vi "lv_list.vi"   [LabVIEW 2020]
doc: "G-CLI tool to list installed LabView development versions.s"
uses:
  <vilib>/Wiresmith Technology/G CLI/Argument Parser/Option Class/Option Configuration.ctl
  <vilib>/Wiresmith Technology/G CLI/Argument Parser/Option Class/Argument Type.ctl
  <vilib>/Utility/error.llb/DialogType.ctl
  094f6021-4ef8-4573-82ce-a7b4949f6c5c.vi
  67a138f0-9744-4b2d-9c21-223ad79f4533.vi
  6795289f-0a04-455c-a499-a5e59a361415.vi
  <vilib>/JDP Science/JSONtext/Variant to JSON Text.vi
  <vilib>/JDP Science/JSONtext/LVClass Serializer/JSONtext LVClass Serializer.lvclass
  <vilib>/regexp/Match Regular Expression.xnode
  <vilib>/Wiresmith Technology/G CLI/CLI Class/CLI.lvclass
  <vilib>/Wiresmith Technology/G CLI/Argument Parser/Option Set Class/Option Set.lvclass
  <vilib>/Wiresmith Technology/G CLI/Argument Parser/Option Class/Option.lvclass
  <vilib>/JDP Science/JSONtext/JSONtext.lvlib
types:
  T1 = cluster{"VerboseMode":bool, "JsonOutput":bool, "ShortOutput":bool}
  T2 = enum32{"Invalid", "Standard", "Closed", "Hidden", "Minimized", "Maximized"}
  T3 = typedef "Option Parser.lvlib/Option.lvclass/Option Configuration.ctl" = cluster{"Option Type":T4, "Option Labels":string[], "Key":string, "Description":string, "Required":bool, "Default Value":string}
  T4 = typedef "Option Parser.lvlib/Option.lvclass/Argument Type.ctl" = enum16{"flag", "value"}
  T5 = typedef "LabViewApplication--cluster.ctl" = cluster{"Bitness":enum8{"Unknown", "x86", "x64"}, "Version":string, "LabVIEW.exe":path, "VersionString":string}
  T6 = typedef "DialogType.ctl" = u16
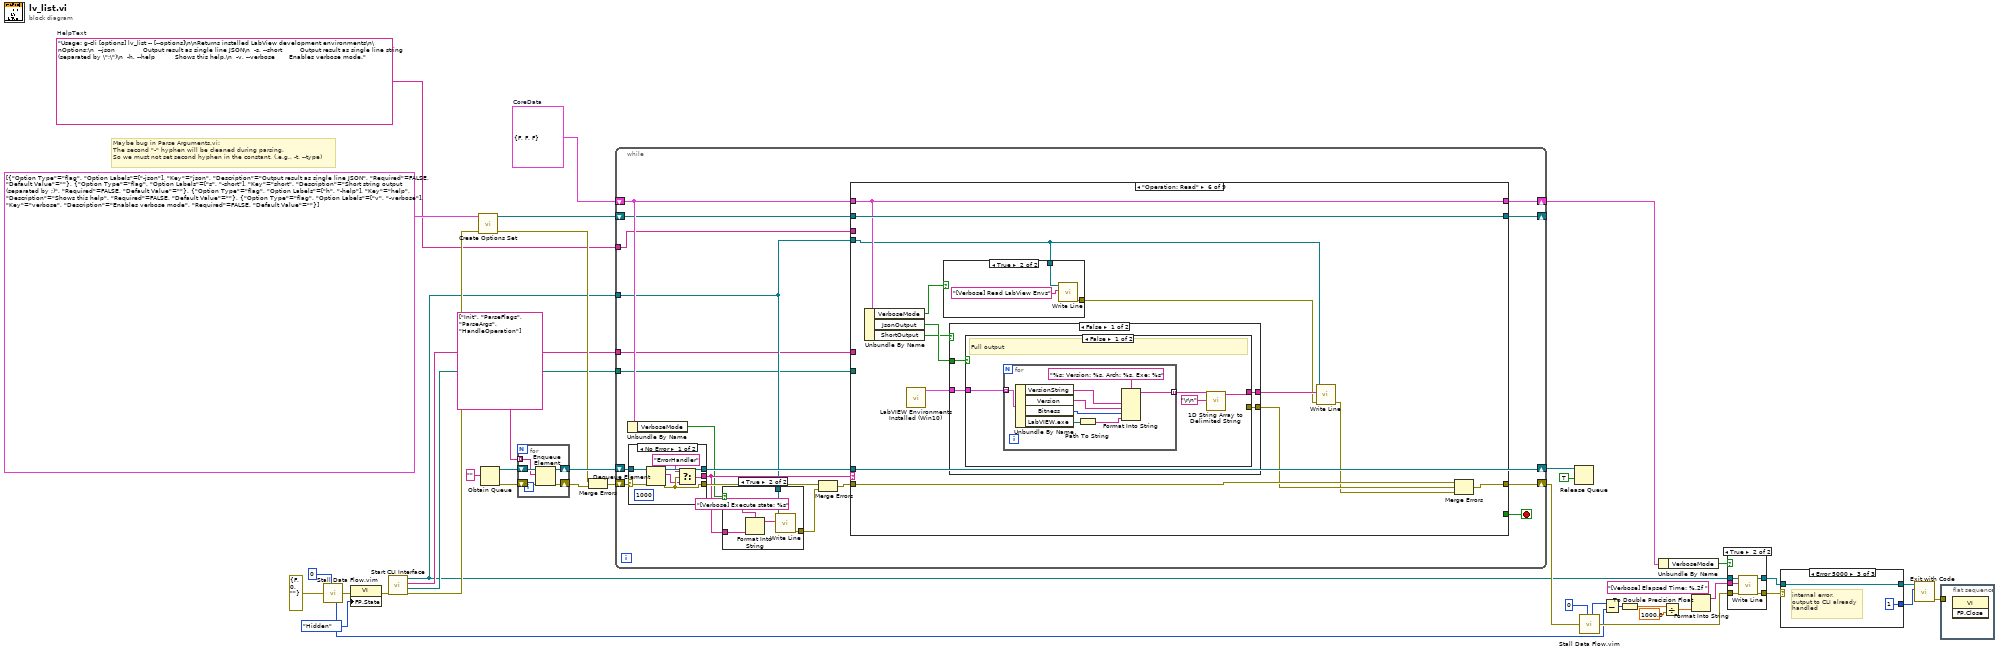
[diagram p0: block diagram]
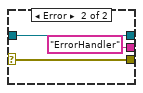
[diagram p4: hidden frame]
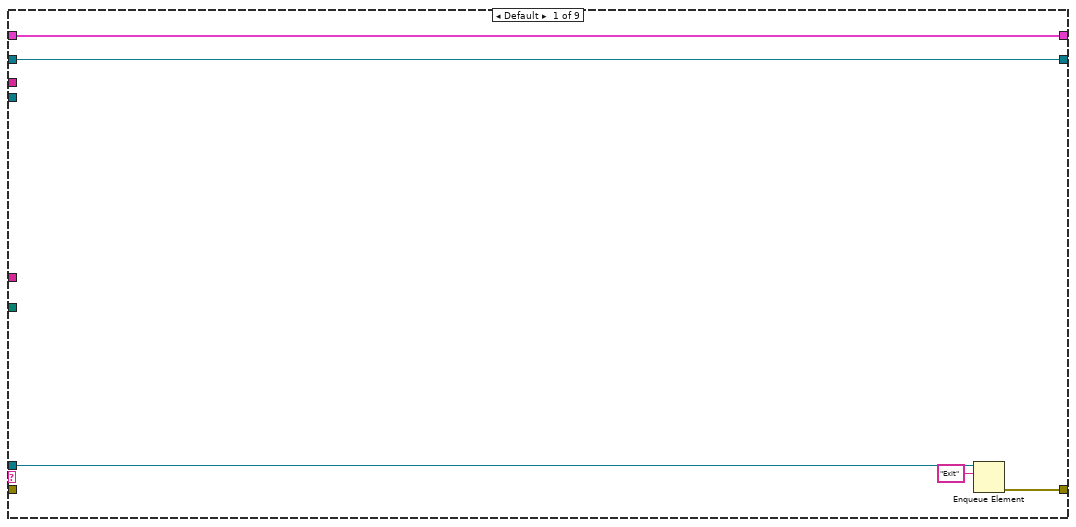
[diagram p5: hidden frame]
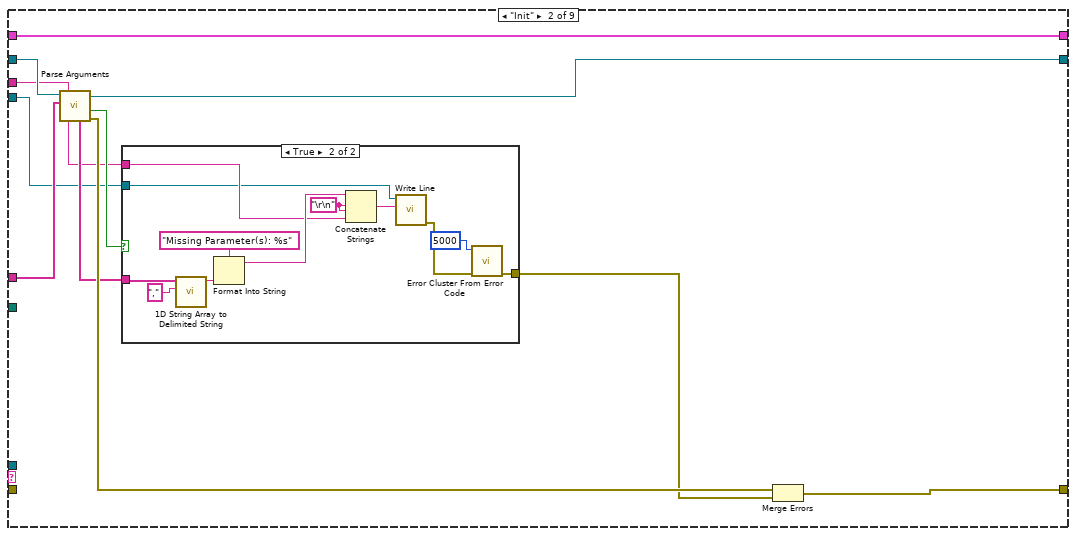
[diagram p6: hidden frame]
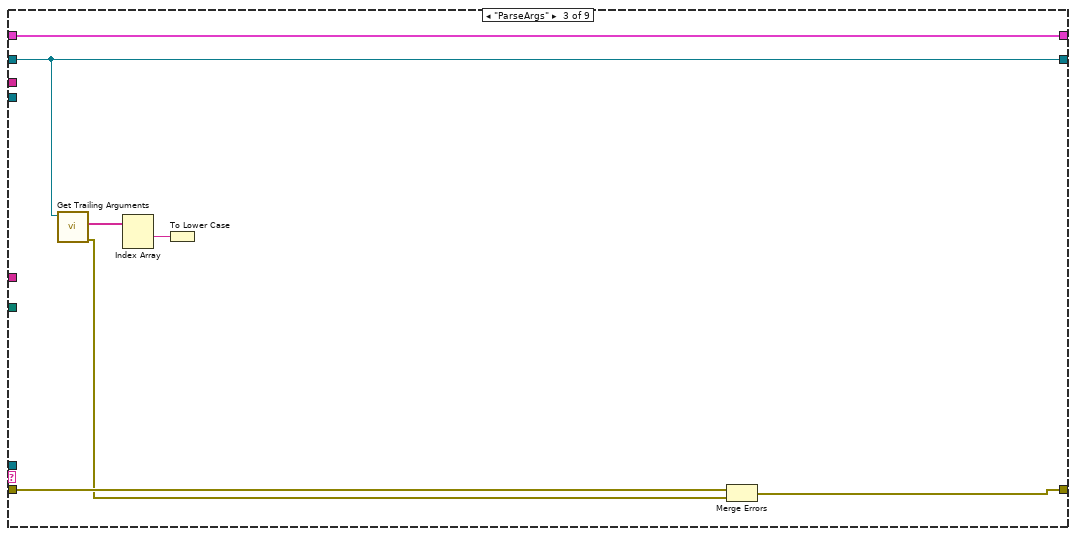
[diagram p8: hidden frame]
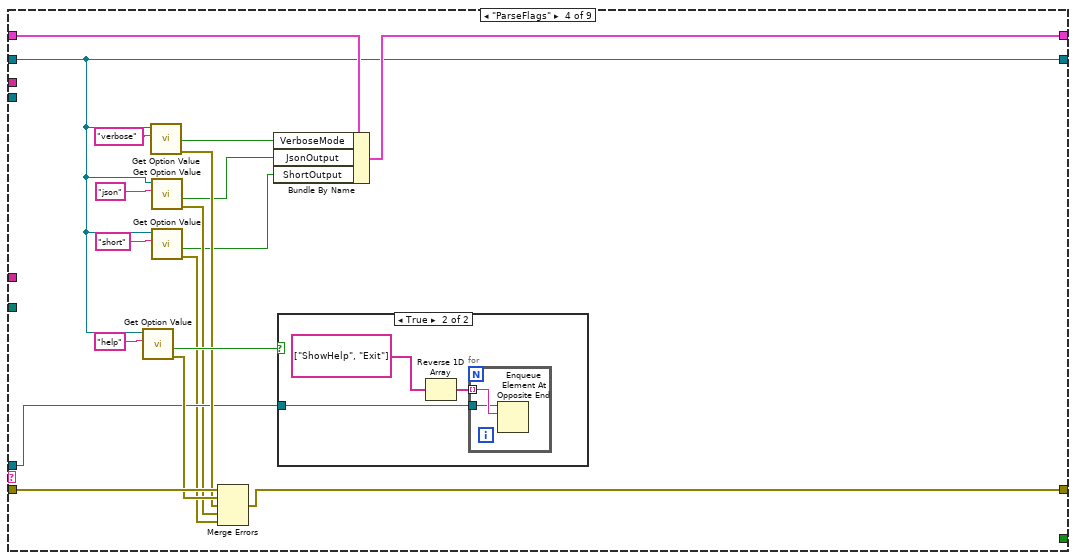
[diagram p9: hidden frame]
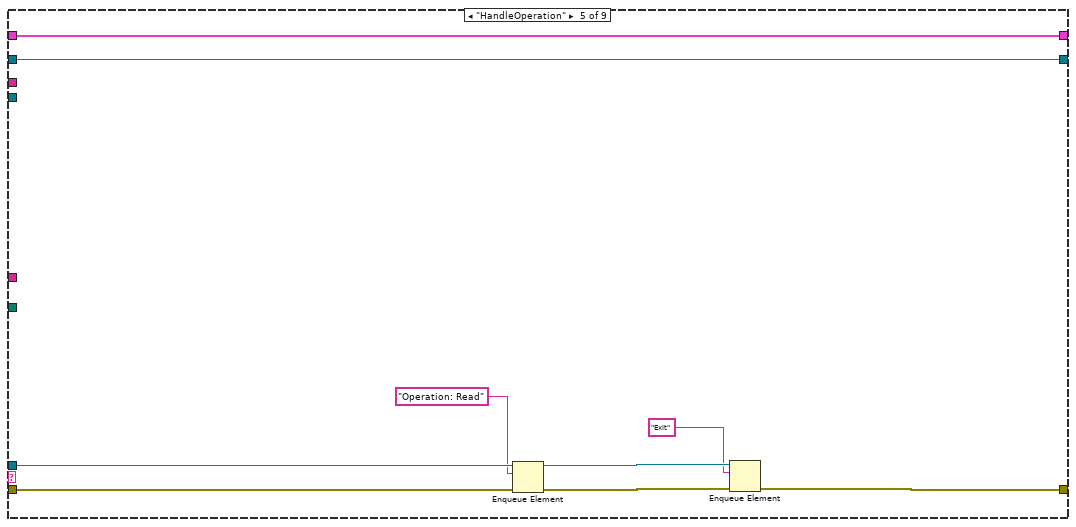
[diagram p11: hidden frame]
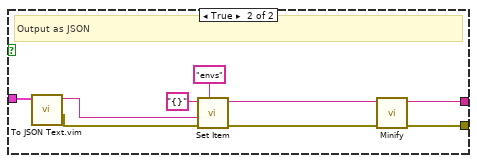
[diagram p12: hidden frame]
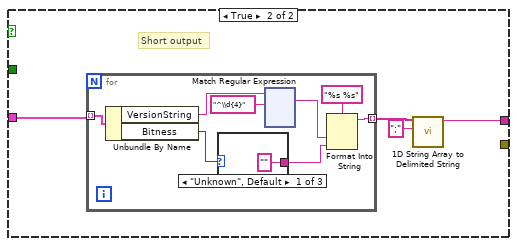
[diagram p13: hidden frame]
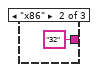
[diagram p14: hidden frame]
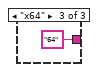
[diagram p15: hidden frame]
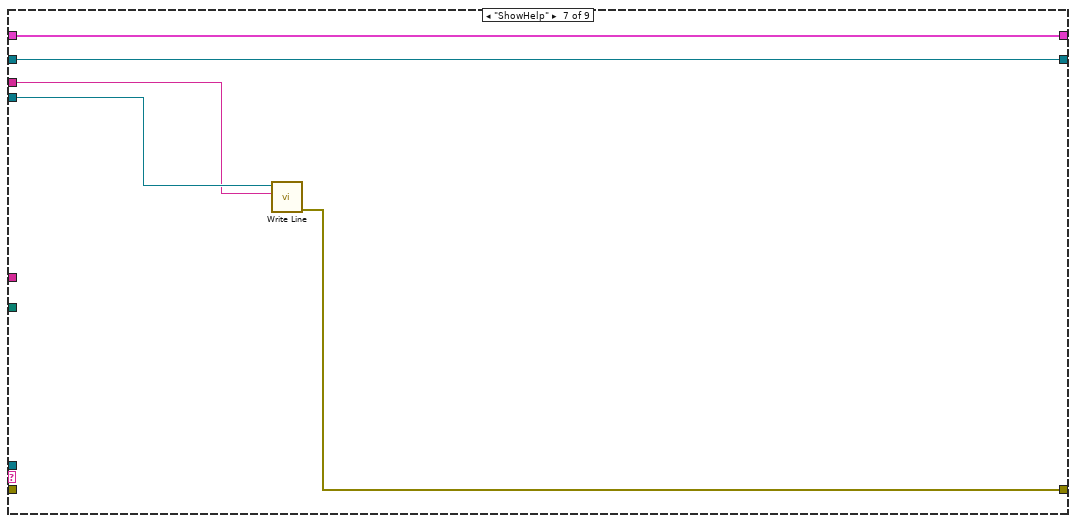
[diagram p17: hidden frame]
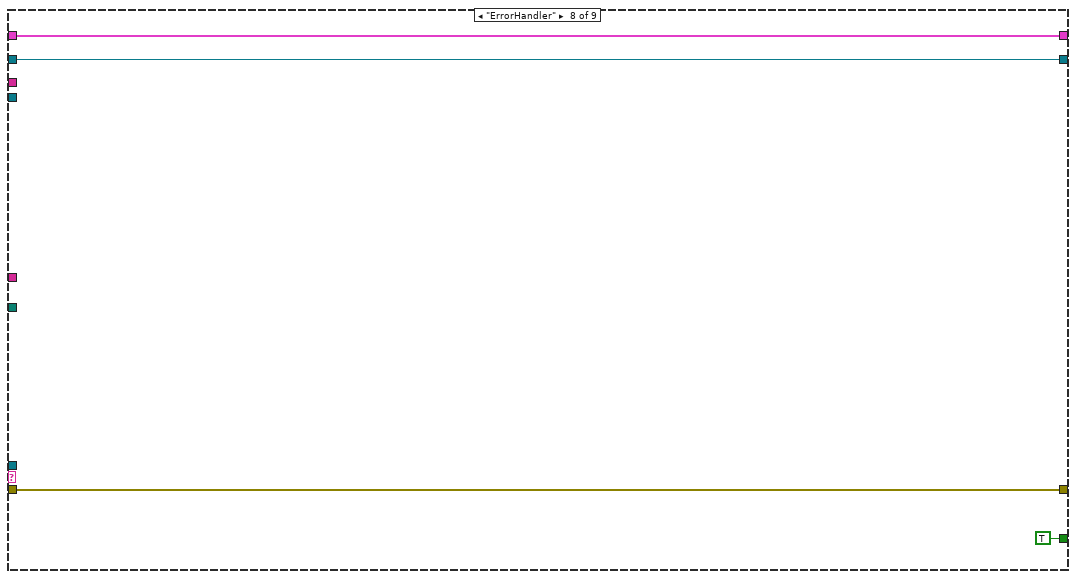
[diagram p18: hidden frame]
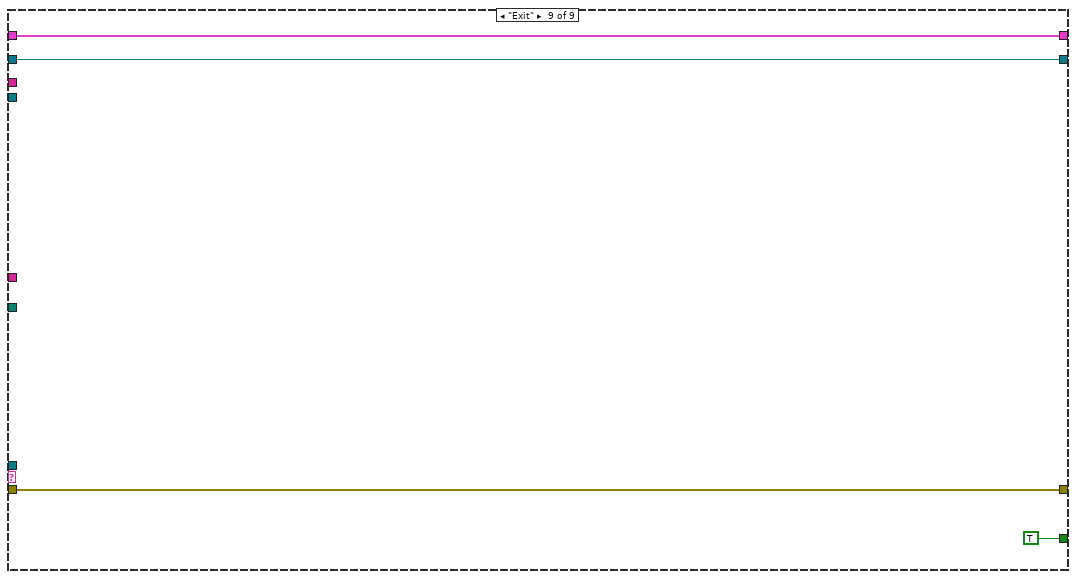
[diagram p19: hidden frame]
diagram:
  w1 = "Usage: g-cli [options] lv_list -- [--options]\n\nReturns installed LabView development environments\n\nOptions:\n  --json              Output result as single line JSON\n  -s, --short         Output result as single line string (separated by \";\")\n  -h, --help          Shows this help.\n  -v, --verbose       Enables verbose mode."  # HelpText
  w14 = T1 {"VerboseMode"=FALSE, "JsonOutput"=FALSE, "ShortOutput"=FALSE}  # CoreData
  # "Maybe bug in Parse Arguments.vi: \nThe second \"-\" hyphen will be cleaned during parsing.\nSo we must not set second hyphen in the constant. (.e.g., -t, --type)"
  n1 = call "Stall Data Flow.vim"("value in"=errorcluster {"status"=FALSE, "code"=0, "source"=""} ("error in (no error)"), "milliseconds to wait"=u32 0) -> ("millisecond timer value"=w30:u32, "value out"=w37:errorcluster)
  n2 = property class="VI"(error in=w37, "FP.State"=T2."Hidden" ("Front Panel Window:State")) -> (error out=w36:errorcluster)  [unwired: 1 in, 1 out]
  n3 = call <vilib>:"Start CLI Interface.vi"("error in (no error)"=w36) -> ("error out"=w41:errorcluster, "Working Directory"=w7:path, "Custom Parameters"=w8:string[], "CLI out"=w5:refnum<class "CLI.lvclass">)  [unwired: 7 in]
  n4 = call <vilib>:"Create Options Set.vi"("error in (no error)"=w41, "Options"=T3[] [{"Option Type"=enum."flag", "Option Labels"=["-json"], "Key"="json", "Description"="Output result as single line JSON", "Required"=FALSE, "Default Value"=""}, {"Option Type"=enum."flag", "Option Labels"=["s", "-short"], "Key"="short", "Description"="Short string output (separated by ;)", "Required"=FALSE, "Default Value"=""}, {"Option Type"=enum."flag", "Option Labels"=["h", "-help"], "Key"="help", "Description"="Shows this help", "Required"=FALSE, "Default Value"=""}, {"Option Type"=enum."flag", "Option Labels"=["v", "-verbose"], "Key"="verbose", "Description"="Enables verbose mode", "Required"=FALSE, "Default Value"=""}]) -> ("error out"=w10:errorcluster, "Option Set out"=w12:refnum<class "Option Set.lvclass">)  [unwired: 8 in]
  n5 = Obtain Queue(element data type="") -> (queue out=w19:refnum<queue>, error out=w16:errorcluster)  [unwired: 4 in, 1 out]
  n6 = for {
    shift-right: [w45] -> w17
    shift-left: w19 -> [w46]
    shift-right: [w43] -> w11
    shift-left: w16 -> [w44]
    tunnel: string[] ["Init", "ParseFlags", "ParseArgs", "HandleOperation"] -> [w42] mode=indexing
    n7 = Enqueue Element(queue=w46, element=w42, error in (no error)=w44) -> (queue out=w45:refnum<queue>, error out=w43:errorcluster)  [unwired: 1 in, 1 out]
  }
  n8 = Merge Errors(w10, w11) -> (w9:errorcluster)
  n9 = while {
    shift-right: [w61] -> w4
    shift-left: w14 -> [w56]
    shift-right: [w59] -> w6
    shift-left: w9 -> [w63]
    shift-right: [w58] -> w15
    shift-left: w17 -> [w64]
    tunnel: w5 -> [w54]
    tunnel: w8 -> [w49]
    tunnel: w7 -> [w50]
    tunnel: w1 -> [w48]
    shift-right: [w47] -> _
    shift-left: w12 -> [w53]
    stop <- w60 stop-if-true
    n10 = Unbundle By Name(w56) -> ("VerboseMode"=w55:bool)
    n11 = case shown="No Error" w63 {
      selector: w63 -> [w75 w79]
      tunnel: w64 -> [w76 w78]
      tunnel: [w71 "ErrorHandler"] -> w57
      tunnel: [w73 w79] -> w62
      tunnel: [w74 w78] -> w58
      frame No Error {
        (unwired) 1000 ("timeout in ms (-1)")
        n12 = Dequeue Element(queue=w76, error in (no error)=w75) -> (queue out=w74:refnum<queue>, element=w72:string, error out=w73:errorcluster)  [unwired: 1 in, 1 out]
        n13 = Select(t="ErrorHandler", s=w73, f=w72) -> (s? t:f=w71:string)
      }
      frame Error {
      }
    }
    n14 = case shown="True" w55 {
      tunnel: w57 -> [_ w69]
      tunnel: w54 -> [_ w66]
      tunnel: [_ w65] -> w51
      frame False {
      }
      frame True {
        n15 = Format Into String(format string="[Verbose] Execute state: %s", w69) -> (resulting string=w67:string)  [unwired: 2 in, 1 out]
        n16 = call <vilib>:"Write Line.vi"("Text to Write"=w67, "CLI in"=w66) -> ("error out"=w65:errorcluster)  [unwired: 8 in, 1 out]
      }
    }
    n17 = Merge Errors(w62, w51) -> (w52:errorcluster)
    n18 = case shown="\"Operation: Read\"" w57 {
      tunnel: w52 -> [_ _ w113 w129 w144 w157 _ w324 w327]
      tunnel: [w84 w95 w114 w122 w145 w158 w321 w325 w329] -> w61
      tunnel: w56 -> [w84 w95 w114 w132 w145 w158 w321 w325 w329]
      tunnel: [_ _ _ _ _ _ _ TRUE TRUE] -> w60
      tunnel: [w82 w87 w109 w127 w139 w156 w317 w324 w327] -> w59
      tunnel: w58 -> [w83 _ _ w123 w143 _ _ _ _]
      tunnel: w54 -> [_ w88 _ _ _ w154 w319 _ _]
      tunnel: w53 -> [w80 w94 w112 w117 w146 w159 w320 w322 w326]
      tunnel: w50 -> [_ _ _ _ _ _ _ _ _]
      tunnel: w49 -> [_ w93 _ _ _ _ _ _ _]
      tunnel: w48 -> [_ w89 _ _ _ _ w318 _ _]
      tunnel: [w80 w85 w112 w117 w146 w159 w320 w322 w326] -> w47
      frame Default {
        n19 = Enqueue Element(queue=w83, element="Exit") -> (error out=w82:errorcluster)  [unwired: 2 in, 2 out]
      }
      frame "Init" {
        n20 = call <vilib>:"Parse Arguments.vi"("Arguments"=w93, "Option Set in"=w94) -> ("error out"=w92:errorcluster, "Missing Options"=w91:bool, "Option Set out"=w85:refnum<class "Option Set.lvclass">, "Missing Option Keys"=w90:string[])  [unwired: 6 in]
        n21 = case shown="True" w91 {
          tunnel: w90 -> [_ w106]
          tunnel: w89 -> [_ w101]
          tunnel: w88 -> [_ w99]
          tunnel: [_ w96] -> w86
          frame False {
          }
          frame True {
            w103 = "\r\n"
            n22 = call <vilib>:"1D String Array to Delimited String.vi"("delimiter"=",", "string array"=w106) -> ("delimited string"=w104:string)  [unwired: 9 in]
            n23 = Format Into String(format string="Missing Parameter(s): %s", w104) -> (resulting string=w102:string)  [unwired: 2 in, 1 out]
            n24 = Concatenate Strings(w102, w103, w103, w101) -> (w100:string)
            n25 = call <vilib>:"Write Line.vi"("Text to Write"=w100, "CLI in"=w99) -> ("error out"=w97:errorcluster)  [unwired: 8 in, 1 out]
            n26 = call <vilib>:"Error Cluster From Error Code.vi"("error in (no error)"=w97, "error code (0)"=5000) -> ("error out"=w96:errorcluster)  [unwired: 7 in]
          }
        }
        n27 = Merge Errors(w92, w86) -> (w87:errorcluster)
      }
      frame "ParseArgs" {
        n28 = call <vilib>:"Get Trailing Arguments.vi"("Option Set in"=w112) -> ("error out"=w108:errorcluster, "Arguments"=w111:string[])  [unwired: 8 in, 1 out]
        n29 = Index Array(array=w111) -> (element #1=w110:string)  [unwired: 2 in, 1 out]
        n30 = To Lower Case(string=w110) -> ()  [unwired: 1 out]
        n31 = Merge Errors(w113, w108) -> (w109:errorcluster)
      }
      frame "ParseFlags" {
        n32 = call <vilib>:"Get Option Value.vi"("Option Key"="help", "Option Set in"=w117) -> ("error out"=w126:errorcluster, "Set"=w130:bool)  [unwired: 6 in, 2 out]
        n33 = call <vilib>:"Get Option Value.vi"("Option Key"="verbose", "Option Set in"=w117) -> ("error out"=w125:errorcluster, "Set"=w124:bool)  [unwired: 6 in, 2 out]
        n34 = call <vilib>:"Get Option Value.vi"("Option Key"="json", "Option Set in"=w117) -> ("error out"=w120:errorcluster, "Set"=w119:bool)  [unwired: 6 in, 2 out]
        n35 = call <vilib>:"Get Option Value.vi"("Option Key"="short", "Option Set in"=w117) -> ("error out"=w116:errorcluster, "Set"=w115:bool)  [unwired: 6 in, 2 out]
        n36 = Merge Errors(w129, w126, w125, w120, w116) -> (w127:errorcluster)
        n37 = Bundle By Name(cluster=w132, "VerboseMode"=w124, "JsonOutput"=w119, "ShortOutput"=w115) -> (w122:T1)
        n38 = case shown="True" w130 {
          tunnel: w123 -> [_ w134]
          frame False {
          }
          frame True {
            n39 = Reverse 1D Array(array=string[] ["ShowHelp", "Exit"]) -> (reversed array=w133:string[])
            n40 = for {
              tunnel: w133 -> [w137] mode=indexing
              tunnel: w134 -> [w136]
              n41 = Enqueue Element At Opposite End(queue=w136, element=w137) -> ()  [unwired: 2 in, 3 out]
            }
          }
        }
      }
      frame "HandleOperation" {
        n42 = Enqueue Element(queue=w143, element="Operation: Read", error in (no error)=w144) -> (queue out=w141:refnum<queue>, error out=w142:errorcluster)  [unwired: 1 in, 1 out]
        n43 = Enqueue Element(queue=w141, element="Exit", error in (no error)=w142) -> (error out=w139:errorcluster)  [unwired: 1 in, 2 out]
      }
      frame "Operation: Read" {
        n44 = Unbundle By Name(w158) -> ("VerboseMode"=w155:bool, "JsonOutput"=w149:bool, "ShortOutput"=w147:bool)
        n45 = call "LabVIEW Environments Installed (Win10).vi"() -> ("LabVIEW Applications Installed"=w153:T5[])  [unwired: 9 in, 2 out]
        n46 = case shown="True" w155 {
          tunnel: w154 -> [_ w316]
          tunnel: [_ w315] -> w148
          frame False {
          }
          frame True {
            n47 = call <vilib>:"Write Line.vi"("Text to Write"="[Verbose] Read LabView Envs" ("format string"), "CLI in"=w316) -> ("error out"=w315:errorcluster)  [unwired: 8 in, 1 out]
          }
        }
        n48 = case shown="False" w147 {
          tunnel: w153 -> [w163 w187]
          tunnel: [w162 _] -> w152
          tunnel: [w161 w188] -> w151
          tunnel: w149 -> [w160 _]
          frame False {
            n49 = case shown="False" w160 {
              tunnel: w163 -> [w167 w184]
              tunnel: [_ w183] -> w162
              tunnel: [w165 w182] -> w161
              frame False {
                # "Full output"
                n50 = for {
                  tunnel: w167 -> [w175] mode=indexing
                  tunnel: [w168] -> w166 mode=indexing
                  n51 = Unbundle By Name(w175) -> ("VersionString"=w170:string, "Version"=w171:string, "Bitness"=w172:enum8{"Unknown", "x86", "x64"}, "LabVIEW.exe"=w174:path)
                  n52 = Path To String(path=w174) -> (string=w173:string)
                  n53 = Format Into String(format string="%s: Version: %s, Arch: %s, Exe: %s", w170, w171, w172, w173) -> (resulting string=w168:string)  [unwired: 2 in, 1 out]
                }
                n54 = call <vilib>:"1D String Array to Delimited String.vi"("delimiter"="\r\n", "string array"=w166) -> ("delimited string"=w165:string)  [unwired: 9 in]
              }
              frame True {
                # "Output as JSON"
                n55 = call "To JSON Text.vim"("Anything"=w184) -> ("error out"=w180:errorcluster, "<JSON>"=w181:string)  [unwired: 9 in]
                n56 = call <vilib>:"Set Item.vi"("$Path or Item Name"="envs", "error in (no error)"=w180, "JSON to Insert"=w181, "JSON"="{}") -> ("error out"=w179:errorcluster, "<JSON>"=w177:string)  [unwired: 4 in, 1 out]
                n57 = call <vilib>:"Minify.vi"("error in (no error)"=w179, "JSON"=w177) -> ("error out"=w183:errorcluster, "<JSON>"=w182:string)  [unwired: 7 in, 1 out]
              }
            }
          }
          frame True {
            # "Short output"
            n58 = for {
              tunnel: w187 -> [w196] mode=indexing
              tunnel: [w189] -> w186 mode=indexing
              n59 = Unbundle By Name(w196) -> ("VersionString"=w195:string, "Bitness"=w193:enum8{"Unknown", "x86", "x64"})
              n60 = case shown="\"Unknown\", Default" w193 {
                tunnel: ["" ("regular expression") "32" ("regular expression") "64" ("regular expression")] -> w190
                frame "Unknown", Default {
                }
                frame "x86" {
                }
                frame "x64" {
                }
              }
              n61 = xnode "Match Regular Expression"("input string"=w195, "regular expression"="^\\d{4}") -> ("whole match"=w191:string)  [unwired: 4 in, 4 out]
              n62 = Format Into String(format string="%s %s", w191, w190) -> (resulting string=w189:string)  [unwired: 2 in, 1 out]
            }
            n63 = call <vilib>:"1D String Array to Delimited String.vi"("delimiter"=";", "string array"=w186) -> ("delimited string"=w188:string)  [unwired: 9 in]
          }
        }
        n64 = call <vilib>:"Write Line.vi"("error in (no error)"=w148, "Text to Write"=w151, "CLI in"=w154) -> ("error out"=w150:errorcluster)  [unwired: 7 in, 1 out]
        n65 = Merge Errors(w157, w152, w150) -> (w156:errorcluster)
      }
      frame "ShowHelp" {
        n66 = call <vilib>:"Write Line.vi"("Text to Write"=w318, "CLI in"=w319) -> ("error out"=w317:errorcluster)  [unwired: 8 in, 1 out]
      }
      frame "ErrorHandler" {
      }
      frame "Exit" {
      }
    }
  }
  n67 = Release Queue(queue=w15, force destroy? (F)=TRUE) -> ()  [unwired: 1 in, 3 out]
  n68 = call "Stall Data Flow.vim"("value in"=w6, "milliseconds to wait"=u32 0) -> ("millisecond timer value"=w31:u32, "value out"=w39:errorcluster)
  n69 = Subtract(x=w31, y=w30) -> (x-y=w29:u32)
  n70 = To Double Precision Float(number=w29) -> (double precision float=w28:dbl)
  n71 = Unbundle By Name(w4) -> ("VerboseMode"=w3:bool)
  n72 = Divide(x=w28, y=1000.0) -> (x/y=w26:dbl)
  n73 = Format Into String(format string="[Verbose] Elapsed Time: %.2f ", w26) -> (resulting string=w24:string)  [unwired: 2 in, 1 out]
  n74 = case shown="True" w3 {
    tunnel: w39 -> [w330 w336]
    tunnel: [w330 w335] -> w38
    tunnel: w5 -> [w331 w334]
    tunnel: w24 -> [_ w333]
    tunnel: [w331 w332] -> w23
    frame False {
    }
    frame True {
      n75 = call <vilib>:"Write Line.vi"("error in (no error)"=w336, "Text to Write"=w333, "CLI in"=w334) -> ("error out"=w335:errorcluster, "CLI out"=w332:refnum<class "CLI.lvclass">)  [unwired: 7 in]
    }
  }
  n76 = case shown="Error 5000" w38 {
    selector: w38 -> [_ w343 _]
    tunnel: w23 -> [w337 w342 w344]
    tunnel: [w337 w341 w344] -> w22
    tunnel: [_ w338 1 ("code out")] -> w21
    frame No Error {
    }
    frame Default {
      w340 = T6 0 items=["no dialog", "OK message", "continue or stop message", "OK message + warnings", "continue/stop + warnings"] ("type of dialog (OK msg:1)")
      n77 = call <vilib>:"Simple Error Handler.vi"("type of dialog (OK msg:1)"=w340, "error in (no error)"=w343) -> ("code out"=w338:i32, "message"=w339:string)  [unwired: 3 in, 3 out]
      n78 = call <vilib>:"Write Line.vi"("Text to Write"=w339, "CLI in"=w342) -> ("CLI out"=w341:refnum<class "CLI.lvclass">)  [unwired: 8 in, 1 out]
    }
    frame Error {
      # "internal error, \noutput to CLI already\nhandled"
    }
  }
  n79 = call <vilib>:"Exit with Code.vi"("Exit Code (0)"=w21, "CLI in"=w22) -> ("error out"=w35:errorcluster)  [unwired: 9 in]
  n80 = flat-sequence {
    tunnel: w35 -> [_]
    frame #0 {
      n81 = invoke class="VI" method="FP.Close"() -> ()  [unwired: 3 in, 3 out]
    }
  }
